vi "GraphChannels.vi"() -> ()   [LabVIEW 2015]
panel:
  in  "2D Array 2":dbl[][](array[numeric])=[[0.0, 0.0], [0.0, 7.0], [7.0, 7.0], [0.0, 0.0]]
  in  "2D Array":dbl[][](array[numeric])=[[0.0, 5.0], [5.0, 5.0], [5.0, 0.0], [7.0, 0.0]]
  out "XY Graph":cluster{"Y":dbl[], "Y":dbl[]}[](graph)=[{"Y"=[0.0, 5.0], "Y"=[0.0, 0.0]}, {"Y"=[5.0, 5.0], "Y"=[0.0, 7.0]}, {"Y"=[5.0, 0.0], "Y"=[7.0, 7.0]}, {"Y"=[7.0, 0.0], "Y"=[0.0, 0.0]}]
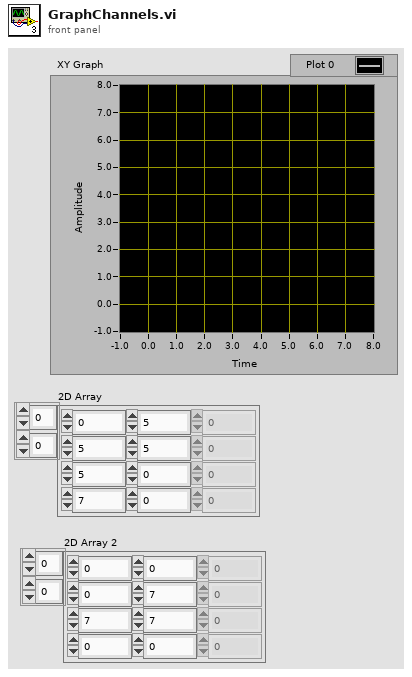
[diagram p1: front panel]
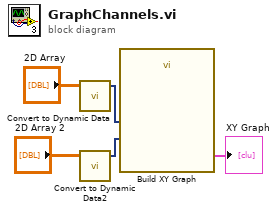
[diagram p0: block diagram]
diagram:
  n1 = call "Convert to Dynamic Data"("2D Array"="2D Array") -> ("Dynamic Data Type"=w3:dynamicdata)  [unwired: 3 in]
  n2 = call "Convert to Dynamic Data2"("2D Array"="2D Array 2") -> ("Dynamic Data Type"=w1:dynamicdata)  [unwired: 3 in]
  n3 = call "Build XY Graph"("Y Input"=w1, "X Input"=w3) -> ("XY Graph"=→"XY Graph":cluster{"X":dbl[], "Y":dbl[]}[])  [unwired: 8 in, 1 out]
